vi "Get Top Level References.vi"(8 "error in (no error)":errorcluster) -> (0 "error out":errorcluster, 2 "Main UI Tab Ref":refnum<vi>, 3 "VI ref":refnum<vi>)   [LabVIEW 2019, in "Configuration Tool.lvlib"]
uses:
  Configuration Tool.lvlib
  <vilib>/Utility/traverseref.llb/TRef TravTarget.ctl
  <vilib>/Utility/traverseref.llb/VI Scripting - Traverse.lvlib
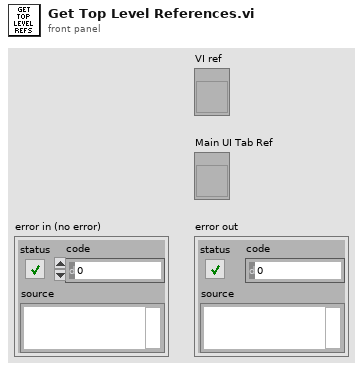
[diagram p1: front panel]
types:
  T1 = typedef "TRef TravTarget.ctl" = enum16{"FP", "BD", "Other"}
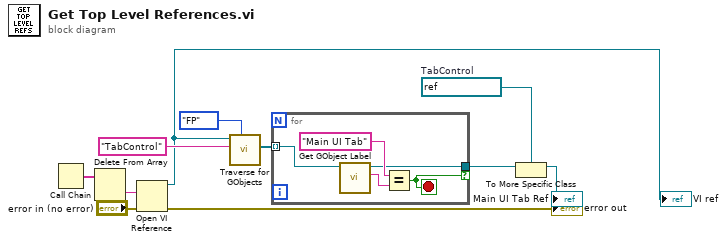
[diagram p0: block diagram]
diagram:
  w8 = refnum<vi> refnum  # TabControl
  n1 = Call Chain() -> (call chain=w2:string[])
  n2 = Delete From Array(array=w2) -> (deleted portion=w3:string)  [unwired: 2 in, 1 out]
  n3 = Open VI Reference(vi path=w3, error in (no error)="error in (no error)") -> (vi reference=w5:refnum<vi>, error out=→"error out":errorcluster)  [unwired: 4 in]
  "VI ref" <- w5
  n4 = call <vilib>:"Traverse for GObjects.vi"("Traverse Target"=TRef_TravTarget."FP", "Class Name"="TabControl", "VI Refnum"=w5) -> ("References"=w10:refnum<vi>[])  [unwired: 5 in, 3 out]
  n5 = for {
    tunnel: w10 -> [w16] mode=indexing
    tunnel: [w13] -> w11 if=w12
    stop <- w12 stop-if-true
    n6 = call <vilib>:"Get GObject Label.vi"("GObject"=w16) -> ("Object Label"=w15:string, "dup GObject"=w13:refnum<vi>)  [unwired: 6 in, 3 out]
    n7 = Equal?(x="Main UI Tab", y=w15) -> (x = y?=w12:bool)
  }
  n8 = To More Specific Class(target class=w8, reference=w11) -> (specific class reference=→"Main UI Tab Ref":refnum<vi>)  [unwired: 1 in, 1 out]
